vi "nanocal -- gradient descent -- V2.vi"(5 "# steps":i32=150, 6 "data":T2={"dz/dω  (sec/rad)"=[], "z "=[1.7183506006211996e-05-0.0001154032788780638i, 1.7124360968751133e-05-0.0001154114779288915i, 1.7049104347380084e-05-0.00011541542942613611i, 1.700437896335042e-05-0.00011541749156201827i, 1.6984579723285106e-05-0.00011542204741013496i, 1.702277369054923e-05-0.00011543195548892015i, 1.713094025845651e-05-0.00011543928112855599i, 1.734249707866828e-05-0.00011543960094139092i, 1.768320429215342e-05-0.0001154245402225022i, 1.8195281152538477e-05-0.00011538335923575508i, 1.8917228661806973e-05-0.00011530288392402138i, 1.9897834564883332e-05-0.00011516640933089982i, 2.154104046962704e-05-0.0001148906117047364i, 2.3247799321765792e-05-0.00011455940834964969i, 2.5364678450551808e-05-0.00011410149936074356i, 2.8645788781885885e-05-0.00011331572480450341i, 3.204749554800641e-05-0.00011242961468546203i, 3.783559691555022e-05-0.00011080033368711338i, 4.245015867332296e-05-0.00010941815048749576i, 4.909131821431355e-05-0.0001073312840925185i, 5.511821898441184e-05-0.00010535829212367013i, 6.178843506022867e-05-0.00010310289174359778i, 7.1079604965352e-05-9.985157907779013e-05i, 7.922304381453334e-05-9.690255343156676e-05i, 8.814778883893872e-05-9.35627973091444e-05i, 9.806709148886077e-05-8.971246458508318e-05i, 0.00011119043245647465-8.437841897470898e-05i, 0.00012253184919712196-7.953180105990741e-05i, 0.00013777724317049346-7.26422052575784e-05i, 0.0001508081004573332-6.638511645494567e-05i, 0.00016547294918783876-5.890291826790314e-05i, 0.00018003847596605868-5.097295421607585e-05i, 0.00019518361086534857-4.2160672625888326e-05i, 0.00021134179818259658-3.207632261667366e-05i, 0.0002372041782935464-1.434566976209705e-05i, 0.00025518143132024254-7.65423157605567e-07i, 0.0002835129702467886+2.297908707067173e-05i, 0.0003060118087631287+4.414715126576145e-05i, 0.00032860772064336976+6.780161699354136e-05i, 0.0003492674091322389+9.188627597766353e-05i, 0.00037498324855458583+0.0001258445655672888i, 0.00040021078021115026+0.00016463936720210011i, 0.00041969942568205823+0.0001996255883353531i, 0.00044367338947118773+0.00025154867300893595i, 0.0004634793607238068+0.0003068834938295352i, 0.00047921028781215815+0.00036805191402776324i, 0.0004880906353641744+0.00042166295770603194i, 0.0004932212623741357+0.0004947057496862386i, 0.000491476456593048+0.0005562791342814882i, 0.000480893803992059+0.0006363872629062725i, 0.0004535995818650303+0.0007373086546111893i, 0.000417087772881063+0.0008226852134031236i, 0.0003564148692854789+0.0009214817173403453i, 0.0003049201646356487+0.0009841224100520793i, 0.00021260191240459413+0.0010684135492785532i, 0.00011714858948470126+0.001130293664798013i, 1.675457544365132e-05+0.0011752384955043165i, -6.8674075405897e-05+0.0012001399159748158i, -0.000156473047607305+0.0012143601357779102i, -0.00026709373934749337+0.0012167952520739987i, -0.0003544271565676041+0.001206585218500233i, -0.00047937600197311275+0.0011721904461218277i, -0.0006086290582260493+0.0011080263068835828i, -0.0007031877411848573+0.0010369948237613604i, -0.0007564526901441745+0.0009845652865779295i, -0.000802489180995596+0.0009292050493656664i, -0.0008414596018105983+0.0008721985101652608i, -0.0008809346482248761+0.0008000538120167723i, -0.0009073902840241921+0.0007382113118499092i, -0.0009264953054508651+0.000680980624166274i, -0.0009405659412141811+0.0006247883223244968i, -0.000951649722530156+0.0005564170049287236i, -0.0009557485581057351+0.0005027508202624884i, -0.0009558464741053665+0.0004515634249715623i, -0.0009509110176922098+0.0003899637122391104i, -0.0009411315169847015+0.00033238768338539245i, -0.0009303400913929496+0.0002890952314710416i, -0.0009171113529290538+0.00024772942260094455i, -0.0009022111527275027+0.00020961974320628598i, -0.0008813746494947608+0.00016554205395646727i, -0.0008581837971946129+0.00012481593212717478i, -0.0008372063466683705+9.328565348151487e-05i, -0.0008165626610594428+6.595676342721183e-05i, -0.0007901155435838691+3.51376371228606e-05i, -0.0007682834352800848+1.2585785624721776e-05i, -0.000746231015527196-7.956667433689733e-06i, -0.0007238798463130141-2.6771164006128246e-05i, -0.0007015567569177018-4.3779400880525094e-05i, -0.000679301954671598-5.9154880569231366e-05i, -0.0006572001413831251-7.301304884663801e-05i, -0.000629855254567978-8.838260380910578e-05i, -0.0006083942229188815-9.917719243438264e-05i, -0.0005768631156754208-0.00011317657292622015i, -0.0005562177438951648-0.00012121832857134644i, -0.0005359092039599222-0.00012831021292074535i, -0.0005145186443378148-0.00013494179211461784i, -0.0004951602053444319-0.00014023403510992087i, -0.00047624970229075174-0.00014478034103386663i, -0.0004577401041527736-0.00014865456703421655i, -0.00043519037796120065-0.00015262867452433312i], "ω (rad/sec)"=[32012.991918577427, 32390.261658505893, 32466.39798177853, 32499.14340521798, 32517.39286113775, 32529.046092051318, 32537.14525712326, 32543.111142615544, 32547.696343954158, 32551.33675949651, 32554.302325209504, 32556.769142360055, 32558.856995237307, 32560.650202739795, 32562.209843476354, 32563.58125099723, 32564.7987833122, 32565.88895894197, 32566.872575330308, 32567.766175404246, 32568.583086316496, 32569.334166794306, 32570.02835688638, 32570.673085530187, 32571.274580490695, 32571.838104118455, 32572.36813539066, 32572.868514009202, 32573.342552524307, 32573.793126289274, 32574.222746575288, 32574.633618125405, 32575.027687968828, 32575.40668442971, 32575.772149741057, 32576.12546690325, 32576.467883345118, 32576.800529469096, 32577.124435064776, 32577.440543590797, 32577.749724325146, 32578.052781957467, 32578.35046682089, 32578.643482565894, 32578.932492128843, 32579.218126471686, 32579.500987779396, 32579.781656707495, 32580.06069600583, 32580.338656060805, 32580.616078519142, 32580.89350097748, 32581.171461032456, 32581.45050033079, 32581.73116925889, 32582.0140305666, 32582.29966469628, 32582.58867447239, 32582.88169000423, 32583.179375080817, 32583.48243271314, 32583.791613234323, 32584.10772197351, 32584.43162756919, 32584.764273480003, 32585.106690135035, 32585.460007297228, 32585.825472395412, 32586.204468856296, 32586.59853891288, 32587.009410462997, 32587.439030535847, 32587.889604513977, 32588.363642815923, 32588.86402143446, 32589.39405291983, 32589.957576334426, 32590.559071508098, 32591.203800151903, 32591.897990030815, 32592.64907072179, 32593.46598163404, 32594.359581707977, 32595.343197883154, 32596.433373726086, 32597.650906041054, 32599.022313348767, 32600.58195429849, 32602.375161800977, 32604.46301467823, 32606.929831615616, 32609.895397541775, 32613.535812870963, 32618.12101442274, 32624.086899701866, 32632.186064986967, 32643.839295900536, 32662.088751820305, 32694.834175046595, 32770.97049853239]}, 7 "action":T3, 8 "newton pars":T4={"newton action"=enum."onlygrads", "weighting"=enum."dω √(|dz/dω|)", "PID-P"=2.328926504017059e-07, "PID-I"=20} {"PID-P" scale=1e-09..1.0 scale format="%#_3p"}, 9 "parameter keys IN":T1[](array[typedef])=[enum."ζ", enum."τ1", enum."τS", enum."τN", enum."τC", enum."κ0"], 10 "parameter Map IN":map{T1, dbl}(c390), 11 "factors Map IN":map{T1, dbl}(c390)) -> (0 "logarithmic derivatives OUT":dbl[](array[numeric])=[-0.0007512892769680174, 0.0016145363736816392, -0.0006397630015226991, 0.02519355182416616, 0.00017978184747877423, -0.00021114437851352735] format="%#_3p", 1 "step factors OUT":map{T1, dbl}(c390), 2 "R(ω) out":cdb[](array[numeric])=[1.7183506006211996e-05+0.0i, 1.7124360968751133e-05+0.0i, 1.7049104347380084e-05+0.0i, 1.700437896335042e-05+0.0i, 1.6984579723285106e-05+0.0i, 1.702277369054923e-05+0.0i, 1.713094025845651e-05+0.0i, 1.734249707866828e-05+0.0i, 1.768320429215342e-05+0.0i, 1.8195281152538477e-05+0.0i, 1.8917228661806973e-05+0.0i, 1.9897834564883332e-05+0.0i, 2.154104046962704e-05+0.0i, 2.3247799321765792e-05+0.0i, 2.5364678450551808e-05+0.0i, 2.8645788781885885e-05+0.0i, 3.204749554800641e-05+0.0i, 3.783559691555022e-05+0.0i, 4.245015867332296e-05+0.0i, 4.909131821431355e-05+0.0i, 5.511821898441184e-05+0.0i, 6.178843506022867e-05+0.0i, 7.1079604965352e-05+0.0i, 7.922304381453334e-05+0.0i, 8.814778883893872e-05+0.0i, 9.806709148886077e-05+0.0i, 0.00011119043245647465+0.0i, 0.00012253184919712196+0.0i, 0.00013777724317049346+0.0i, 0.0001508081004573332+0.0i, 0.00016547294918783876+0.0i, 0.00018003847596605868+0.0i, 0.00019518361086534857+0.0i, 0.00021134179818259658+0.0i, 0.0002372041782935464+0.0i, 0.00025518143132024254+0.0i, 0.0002835129702467886+0.0i, 0.0003060118087631287+0.0i, 0.00032860772064336976+0.0i, 0.0003492674091322389+0.0i, 0.00037498324855458583+0.0i, 0.00040021078021115026+0.0i, 0.00041969942568205823+0.0i, 0.00044367338947118773+0.0i, 0.0004634793607238068+0.0i, 0.00047921028781215815+0.0i, 0.0004880906353641744+0.0i, 0.0004932212623741357+0.0i, 0.000491476456593048+0.0i, 0.000480893803992059+0.0i, 0.0004535995818650303+0.0i, 0.000417087772881063+0.0i, 0.0003564148692854789+0.0i, 0.0003049201646356487+0.0i, 0.00021260191240459413+0.0i, 0.00011714858948470126+0.0i, 1.675457544365132e-05+0.0i, -6.8674075405897e-05+0.0i, -0.000156473047607305+0.0i, -0.00026709373934749337+0.0i, -0.0003544271565676041+0.0i, -0.00047937600197311275+0.0i, -0.0006086290582260493+0.0i, -0.0007031877411848573+0.0i, -0.0007564526901441745+0.0i, -0.000802489180995596+0.0i, -0.0008414596018105983+0.0i, -0.0008809346482248761+0.0i, -0.0009073902840241921+0.0i, -0.0009264953054508651+0.0i, -0.0009405659412141811+0.0i, -0.000951649722530156+0.0i, -0.0009557485581057351+0.0i, -0.0009558464741053665+0.0i, -0.0009509110176922098+0.0i, -0.0009411315169847015+0.0i, -0.0009303400913929496+0.0i, -0.0009171113529290538+0.0i, -0.0009022111527275027+0.0i, -0.0008813746494947608+0.0i, -0.0008581837971946129+0.0i, -0.0008372063466683705+0.0i, -0.0008165626610594428+0.0i, -0.0007901155435838691+0.0i, -0.0007682834352800848+0.0i, -0.000746231015527196+0.0i, -0.0007238798463130141+0.0i, -0.0007015567569177018+0.0i, -0.000679301954671598+0.0i, -0.0006572001413831251+0.0i, -0.000629855254567978+0.0i, -0.0006083942229188815+0.0i, -0.0005768631156754208+0.0i, -0.0005562177438951648+0.0i, -0.0005359092039599222+0.0i, -0.0005145186443378148+0.0i, -0.0004951602053444319+0.0i, -0.00047624970229075174+0.0i, -0.0004577401041527736+0.0i, -0.00043519037796120065+0.0i], 3 "goodness OUT":dbl=0.0013215492647050493 format="%#_3p", 4 "oscillations":cluster{"Array":i32[], "Array":dbl[]})   [LabVIEW 2021]
uses:
  3-lorentzian-parameters.ctl
  nanocal -- gradient descent -- parameters.ctl
  3-lorentzian-heat-response action.ctl
  nanocal-goodness-weighting-strategy.ctl
  nanocal -- gradient descent -- action.ctl
  nanocal -- gradient descent-- data.ctl
  agregator -- action.ctl
  interpolation state - real.ctl
  linear interpolation - real -- V2.vi
  array -- 3-finitediff.vi
  5-lorentzian-heat-response -- analytic derivatives -- grad and curvature -- V6.vi
panel:
  in  "parameter tensor order":map{i32, T1}(c390)
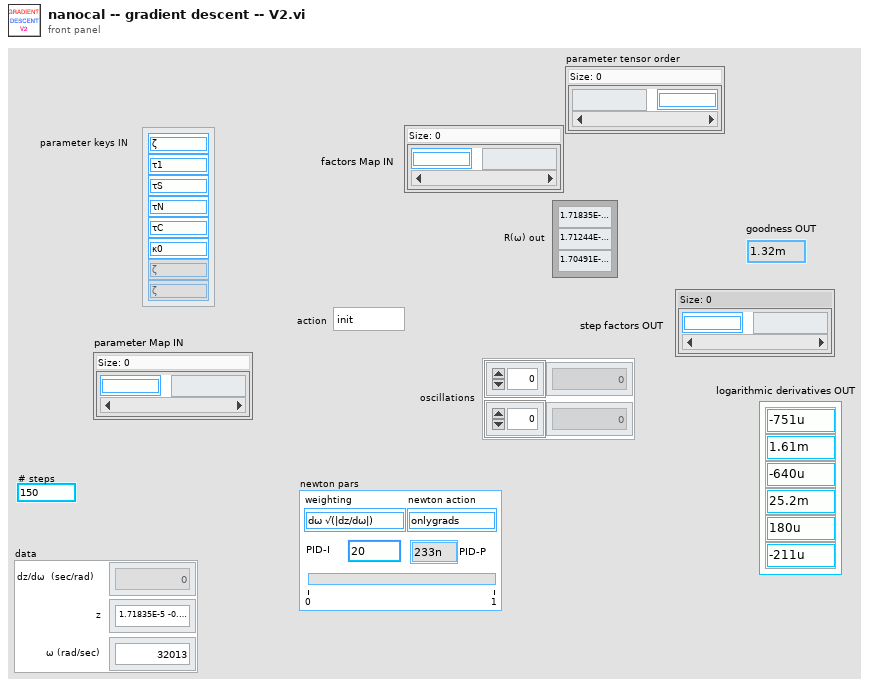
[diagram p1: front panel]
types:
  T1 = typedef "3-lorentzian-parameters.ctl" = enum16{"ζ", "τ1", "τS", "τN", "τC", "κ0", "m1", "m2", "m3", "T (K)", "B (T)", "θ (deg)", "side (S|R)", "set of (B|T)", "Re(offset)", "Im(offset)", "στ1", "στ1-", "στ1+", "στS", "στS-", "στS+", "στN", "στN-", "στN+", "τ11", "τ12", "τ21", "τ22", "τN1", "τN2"}
  T2 = typedef "nanocal -- gradient descent-- data.ctl" = cluster{"dz/dω  (sec/rad)":cdb[], "z ":cdb[], "ω (rad/sec)":dbl[]}
  T3 = typedef "nanocal -- gradient descent -- action.ctl" = enum16{"init", "step", "peek", "sim2nd"}
  T4 = typedef "nanocal -- gradient descent -- parameters.ctl" = cluster{"newton action":T5, "weighting":T6, "PID-P":dbl, "PID-I":i32}
  T5 = typedef "3-lorentzian-heat-response action.ctl" = enum16{"calc R", "create string", "calc m1m2m3", "dζ", "dT1", "dτS", "dτN", "dτC", "d-all", "dκ0", "T(K)", "m1", "m2", "m3", "parse string", "θ (deg)", "B (T)", "onlygrads", "newton", "create emty string", "simple2nd", "calc R2", "ScalarProd", "ScalarProd-diff", "nothing", "ScalarProd-eta"}
  T6 = typedef "nanocal-goodness-weighting-strategy.ctl" = enum16{"dω", "dω √(|dz/dω|)", "dω |dz/dω|", "phase", "andreas", "sum", "anti-andr", "ark"}
  T7 = typedef "agregator -- action.ctl" = enum16{"append", "interpolate", "empty!", "force", "init", "scale", "read last"}
  T8 = typedef "interpolation state - real.ctl" = cluster{"Array ":dbl[], "actual size":i32, "requested size":i32}
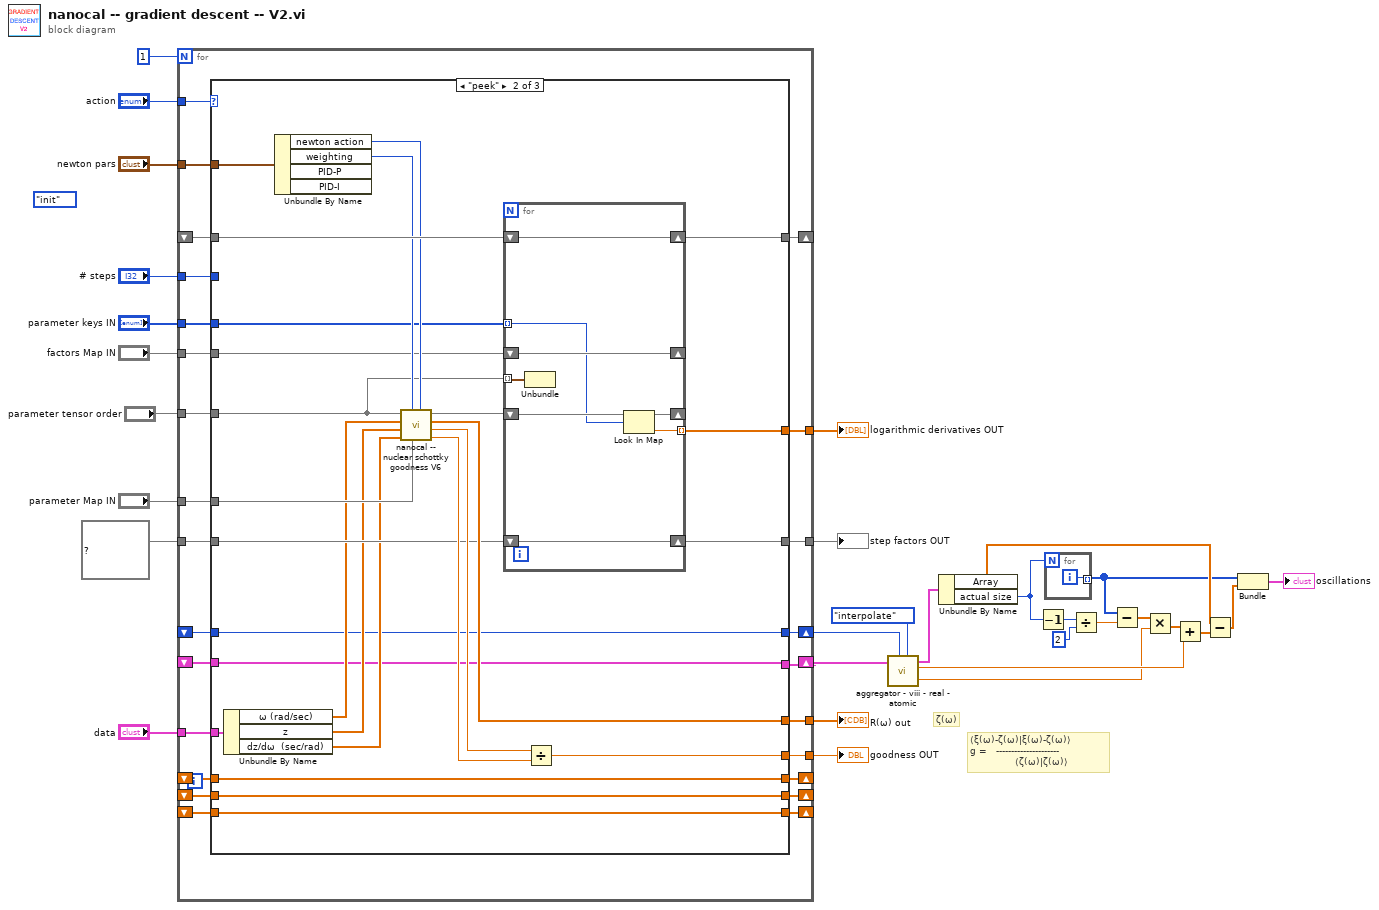
[diagram p0: block diagram]
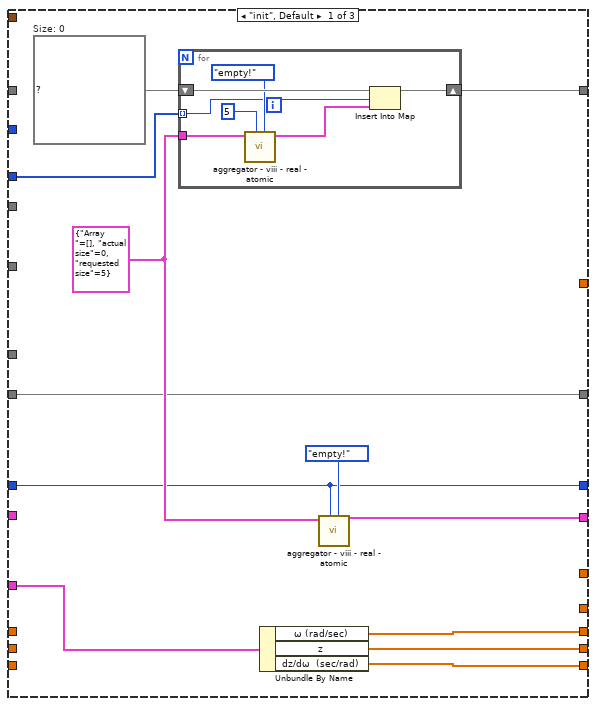
[diagram p2: hidden frame]
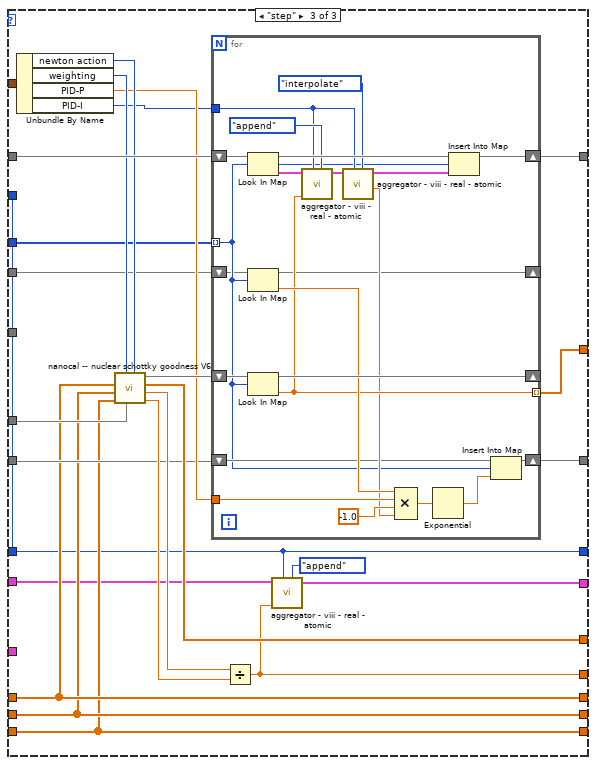
[diagram p3: hidden frame]
diagram:
  (unwired) nanocal_--_gradient_descent_--_action."init" ("action 2")
  # "ζ(ω)"
  # "⟨ξ(ω)-ζ(ω)|ξ(ω)-ζ(ω)⟩ \ng =   ---------------------\n               ⟨ζ(ω)|ζ(ω)⟩"
  n1 = for {
    N: 1 -> [_]
    shift-right: [w52] -> _
    shift-left: _ -> [w53]
    tunnel: "parameter keys IN" -> [w51]
    tunnel: "newton pars" -> [w50]
    tunnel: [w49] -> w28
    tunnel: [w48] -> w27
    tunnel: [w47] -> w26
    tunnel: [w46] -> w25
    tunnel: "parameter Map IN" -> [w45]
    tunnel: "factors Map IN" -> [w44]
    tunnel: map{T1, dbl} {} ("Map IN") -> [w43]
    tunnel: "action" -> [w42]
    shift-right: [w41] -> _
    shift-left: _ -> [w54]
    shift-right: [w40] -> _
    shift-left: _ -> [w55]
    shift-right: [w39] -> _
    shift-left: _ -> [w56]
    tunnel: "data" -> [w38]
    shift-right: [w37] -> w18
    shift-left: _ -> [w36]
    shift-right: [w34] -> w17
    shift-left: _ -> [w35]
    tunnel: "# steps" -> [w33]
    tunnel: "parameter tensor order" -> [w32]
    n2 = case shown="\"peek\"" w42 {
      tunnel: w56 -> [_ w84 w114]
      tunnel: w55 -> [_ w85 w115]
      tunnel: w54 -> [_ w86 w116]
      tunnel: w53 -> [_ w98 w130]
      tunnel: [w63 w97 w129] -> w52
      tunnel: w51 -> [w62 w76 w124]
      tunnel: w50 -> [_ w94 w123]
      tunnel: [_ w93 w110] -> w49
      tunnel: [_ w92 w122] -> w48
      tunnel: [w58 w91 w121] -> w47
      tunnel: [_ w90 w120] -> w46
      tunnel: w45 -> [_ w89 w119]
      tunnel: w44 -> [_ w88 w118]
      tunnel: w43 -> [w58 w87 w117]
      tunnel: [w67 w86 w116] -> w41
      tunnel: [w66 w85 w115] -> w40
      tunnel: [w65 w84 w114] -> w39
      tunnel: w38 -> [w68 w83 _]
      tunnel: [w60 w79 w111] -> w37
      tunnel: w36 -> [_ w79 w112]
      tunnel: w35 -> [w57 w78 _]
      tunnel: [w57 w78 w109] -> w34
      tunnel: w33 -> [_ _ w109]
      tunnel: w32 -> [_ w77 _]
      frame "init", Default {
        w59 = T8 {"Array "=[], "actual size"=0, "requested size"=5} ("Cluster")
        w64 = map{T1, T8} {}  # Size: 0
        n3 = for {
          shift-right: [w74] -> w63
          shift-left: w64 -> [w75]
          tunnel: w62 -> [w71] mode=indexing
          tunnel: w59 -> [w70]
          n4 = call "aggregator - viii - real - atomic.vi"("aggregator action"=agregator_--_action."empty!", "requested size"=5, "state IN"=w70) -> ("state OUT"=w72:T8)  [unwired: 5 in, 3 out]
          n5 = Insert Into Map(map in=w75, key=w71, value=w72) -> (map out=w74:map{T1, T8})  [unwired: 2 out]
        }
        n6 = Unbundle By Name(w68) -> ("ω (rad/sec)"=w67:dbl[], "z"=w66:cdb[], "dz/dω  (sec/rad)"=w65:cdb[])
        n7 = call "aggregator - viii - real - atomic.vi"("aggregator action"=agregator_--_action."empty!", "requested size"=w57, "state IN"=w59) -> ("state OUT"=w60:T8)  [unwired: 5 in, 3 out]
      }
      frame "peek" {
        n8 = Unbundle By Name(w83) -> ("ω (rad/sec)"=w82:dbl[], "z"=w81:cdb[], "dz/dω  (sec/rad)"=w80:cdb[])
        n9 = Unbundle By Name(w94) -> ("newton action"=w96:T5, "weighting"=w95:T6)  [unwired: 2 out]
        n10 = call "nanocal -- nuclear schottky goodness V6.vi"("action"=w96, "parameters IN"=w89, "weighting strategy"=w95, "dz/dω IN (V)"=w80, "ξ(ω) IN (V)"=w81, "ω (rad/sec)"=w82, "parameter tensor order"=w77) -> ("⟨ζ(ω)|ζ(ω)⟩"=w99:dbl, "G = ⟨ξ(ω)|ξ(ω)⟩"=w100:dbl, "|ζ(ω)⟩ out"=w92:cdb[], "dG / dlog λ  =  ⟨ξ(ω) | λdζ(ω)/dλ ⟩"=w101:map{T1, dbl})  [unwired: 1 out]
        n11 = for {
          shift-right: [w108] -> _
          shift-left: w101 -> [w108]
          tunnel: [w106] -> w90 mode=indexing
          shift-right: [w105] -> w97
          shift-left: w98 -> [w105]
          shift-right: [w104] -> w91
          shift-left: w87 -> [w104]
          shift-right: [w107] -> _
          shift-left: w88 -> [w107]
          tunnel: w77 -> [w103] mode=indexing
          tunnel: w76 -> [w102] mode=indexing
          n12 = Unbundle(w103) -> ()  [unwired: 2 out]
          n13 = Look In Map(map=w108, key=w102) -> (value=w106:dbl)  [unwired: 1 in, 1 out]
        }
        n14 = Divide(x=w100, y=w99) -> (x/y=w93:dbl)
      }
      frame "step" {
        n15 = Unbundle By Name(w123) -> ("newton action"=w128:T5, "weighting"=w127:T6, "PID-P"=w126:dbl, "PID-I"=w125:i32)
        n16 = call "nanocal -- nuclear schottky goodness V6.vi"("action"=w128, "parameters IN"=w119, "weighting strategy"=w127, "dz/dω IN (V)"=w114, "ξ(ω) IN (V)"=w115, "ω (rad/sec)"=w116) -> ("⟨ζ(ω)|ζ(ω)⟩"=w131:dbl, "G = ⟨ξ(ω)|ξ(ω)⟩"=w132:dbl, "|ζ(ω)⟩ out"=w122:cdb[], "dG / dlog λ  =  ⟨ξ(ω) | λdζ(ω)/dλ ⟩"=w133:map{T1, dbl})  [unwired: 1 in, 1 out]
        n17 = for {
          tunnel: w124 -> [w135] mode=indexing
          shift-right: [w153] -> _
          shift-left: w133 -> [w153]
          tunnel: [w145] -> w120 mode=indexing
          tunnel: w126 -> [w151]
          shift-right: [w147] -> w129
          shift-left: w130 -> [w148]
          tunnel: w125 -> [w141]
          shift-right: [w138] -> w121
          shift-left: w117 -> [w139]
          shift-right: [w134] -> _
          shift-left: w118 -> [w134]
          n18 = Look In Map(map=w148, key=w135) -> (value=w149:T8)  [unwired: 1 in, 1 out]
          n19 = Look In Map(map=w134, key=w135) -> (value=w150:dbl)  [unwired: 1 in, 1 out]
          n20 = Look In Map(map=w153, key=w135) -> (value=w145:dbl)  [unwired: 1 in, 1 out]
          n21 = call "aggregator - viii - real - atomic.vi"("aggregator action"=agregator_--_action."append", "requested size"=w141, "number"=w145, "state IN"=w149) -> ("state OUT"=w144:T8)  [unwired: 4 in, 3 out]
          n22 = call "aggregator - viii - real - atomic.vi"("aggregator action"=agregator_--_action."interpolate", "requested size"=w141, "state IN"=w144) -> ("interp average"=w143:dbl, "state OUT"=w142:T8)  [unwired: 5 in, 2 out]
          n23 = Compound Arithmetic op=MULTIPLY(w150, w151, -1.0 ("index"), w143) -> (w137:dbl)
          n24 = Exponential(1:w137) -> (0:w136:dbl)
          n25 = Insert Into Map(map in=w148, key=w135, value=w142) -> (map out=w147:map{T1, T8})  [unwired: 2 out]
          n26 = Insert Into Map(map in=w139, key=w135, value=w136) -> (map out=w138:map{T1, dbl})  [unwired: 2 out]
        }
        n27 = Divide(x=w132, y=w131) -> (x/y=w110:dbl)
        n28 = call "aggregator - viii - real - atomic.vi"("aggregator action"=agregator_--_action."append", "requested size"=w109, "number"=w110, "state IN"=w112) -> ("state OUT"=w111:T8)  [unwired: 4 in, 3 out]
      }
    }
  }
  "goodness OUT" <- w28
  "R(ω) out" <- w27
  "step factors OUT" <- w26
  "logarithmic derivatives OUT" <- w25
  n29 = call "aggregator - viii - real - atomic.vi"("aggregator action"=agregator_--_action."interpolate", "requested size"=w17, "state IN"=w18) -> ("slope"=w2:dbl, "mean"=w12:dbl, "state OUT"=w16:T8)  [unwired: 5 in, 1 out]
  n30 = Unbundle By Name(w16) -> ("Array"=w8:dbl[], "actual size"=w11:i32)
  n31 = Decrement(x=w11) -> (x-1=w15:i32)
  n32 = for {
    N: w11 -> [_]
    tunnel: [w154] -> w7 mode=indexing
    i -> [w154]
  }
  n33 = Divide(x=w15, y=2) -> (x/y=w10:dbl)
  n34 = Subtract(x=w7, y=w10) -> (x-y=w3:dbl[])
  n35 = Multiply(x=w3, y=w2) -> (x*y=w13:dbl[])
  n36 = Add(x=w13, y=w12) -> (x+y=w9:dbl[])
  n37 = Subtract(x=w8, y=w9) -> (x-y=w6:dbl[])
  n38 = Bundle(w7, w6) -> (→"oscillations":cluster{i32[], dbl[]})  [unwired: 1 in]
